vi "MB ICPCON Param Read Ip addrs.vi"(8 "error in (no error)":errorcluster, 9 "Lenght (1)":i32, 10 "N (0)":i32, 11 "Param Reference in":T1) -> (0 "error out":errorcluster, 1 "IP address":T2(array[cluster]), 3 "Param Reference out":T1)   [LabVIEW 2021, in "ICPCON_Param.lvlib"]
uses:
  ICPCON_Param.lvlib
  ICPCON Param.ctl
  Eth timeouts.ctl
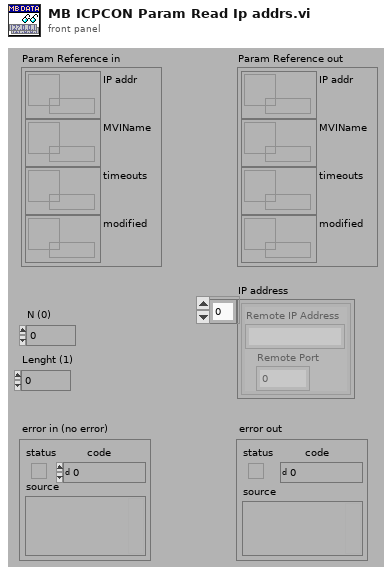
[diagram p1: front panel]
types:
  T1 = typedef "ICPCON_Param.lvlib/ICPCON Param.ctl" = cluster{"IP addr":refnum<data-value>, "MVIName":refnum<data-value>, "timeouts":refnum<data-value>, "modified":refnum<data-value>}
  T2 = cluster{"Remote IP Address":string, "Remote Port":u16}[]
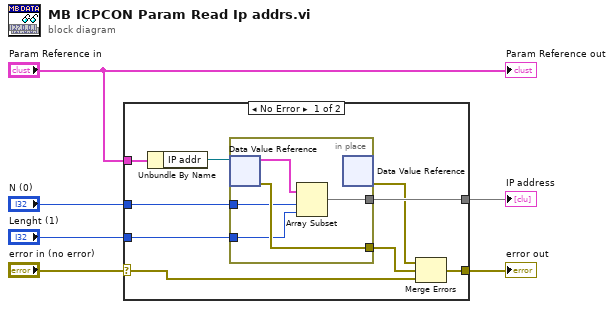
[diagram p0: block diagram]
diagram:
  n1 = case shown="No Error" "error in (no error)" {
    selector: "error in (no error)" -> [w7 w21]
    tunnel: [w12 w21] -> w6
    tunnel: [w15 _] -> w4
    tunnel: "N (0)" -> [w14 _]
    tunnel: "Param Reference in" -> [w13 _]
    tunnel: "Lenght (1)" -> [w9 _]
    frame No Error {
      n2 = Unbundle By Name(w13) -> ("IP addr"=w8:refnum<data-value>)
      n3 = in-place {
        in-place-border: w14 -> [w18]
        in-place-border: [w17] -> w15
        in-place-border: [w20] -> w10
        in-place-border: w9 -> [w16]
        n4 = in-place-dvr #1(w8) -> (w19:T2, w20:errorcluster)
        n5 = Array Subset(array=w19, index=w18, length=w16) -> (w17:T2)
        n6 = in-place-dvr #1() -> (w11:errorcluster)  [unwired: 1 in, 1 out]
      }
      n7 = Merge Errors(w11, w10, w7) -> (w12:errorcluster)
    }
    frame Error {
    }
  }
  "error out" <- w6
  "IP address" <- w4
  "Param Reference out" <- "Param Reference in"
